vi "SubVI-AOMvolt-Power Calibration for 1064-PDver.vi"(3 "milliseconds to wait":u32=200, 4 "scan step #":dbl=25.0, 5 "Max voltage (V)":dbl=4.000000000000001, 6 "Min voltage (V)":dbl=0.5) -> (1 "Polynomial Coefficients":dbl[](array[numeric]) format="%0.2f", 2 "output cluster":T1)   [LabVIEW 2014]
uses:
  <vilib>/Analysis/baseanly.llb/Mean (DBL).vi
  <vilib>/Utility/file.llb/Write To Spreadsheet File (DBL).vi
  <vilib>/Analysis/NI_AALPro.lvlib
  <vilib>/Analysis/NI_AALBase.lvlib
panel:
  out "Cal-PD (mV)":dbl[](array[numeric])
  out "Cal-AOM (V)":dbl[](array[numeric])
  out "PD-AOM Graph":T2(graph)
  out "Voltage to AOM (V)":dbl
  out "Photodiode readout (mV)":dbl
  out "Scan size per step (V)":dbl=0.25
  in  "save cal curve?":bool
  # "**activate \ncontinuous power\ncontinuous AOM"
  # "continuous scaning power \nover AOM voltage range"
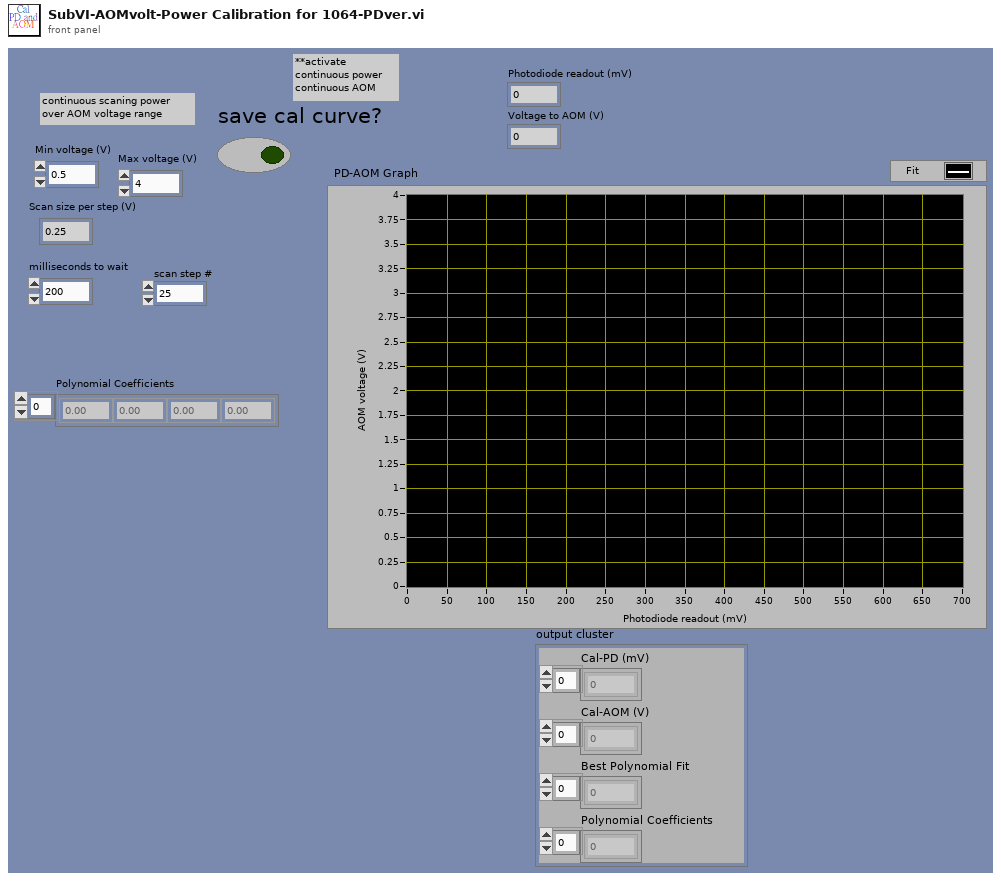
[diagram p1: front panel]
types:
  T1 = cluster{"Cal-PD (mV)":dbl[], "Cal-AOM (V)":dbl[], "Best Polynomial Fit":dbl[], "Polynomial Coefficients":dbl[]}
  T2 = cluster{"Cal-PD (mV)":dbl[], "Cal-AOM (V)":dbl[]}[]
  T3 = cluster{"Cal-PD (mV)":dbl[], "Best Polynomial Fit":dbl[]}
  T4 = cluster{"Cal-PD (mV)":dbl[], "Cal-AOM (V)":dbl[]}
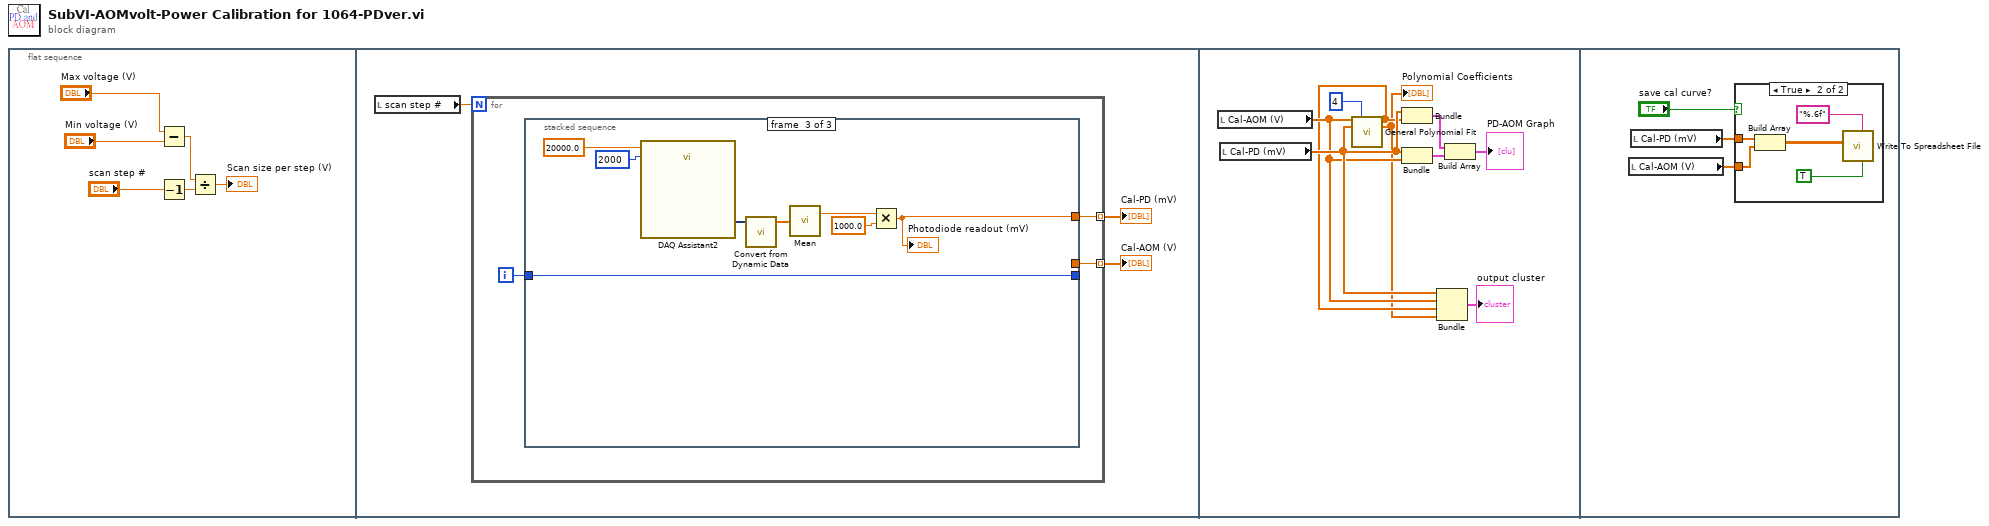
[diagram p0: block diagram]
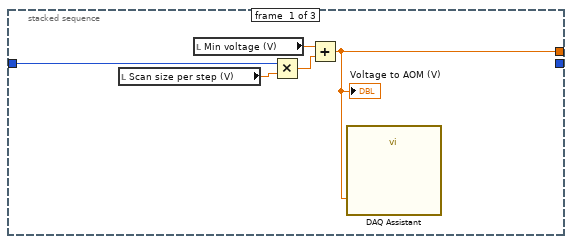
[diagram p2: hidden frame]
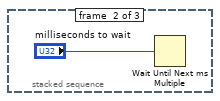
[diagram p3: hidden frame]
diagram:
  n1 = flat-sequence {
    frame #0 {
      n2 = Subtract(x="Max voltage (V)", y="Min voltage (V)") -> (x-y=w3:dbl)
      n3 = Decrement(x="scan step #") -> (x-1=w5:dbl)
      n4 = Divide(x=w3, y=w5) -> (x/y=→"Scan size per step (V)":dbl)
    }
    frame #1 {
      n5 = local read "scan step #"() -> (w9:dbl)
      n6 = for {
        N: w9 -> [_]
        tunnel: [w11] -> w7 mode=indexing
        tunnel: [w10] -> w8 mode=indexing
        i -> [w12]
        n7 = stacked-sequence {
          tunnel: w12 -> [w14 _ w26]
          tunnel: [_ _ w26] -> _
          tunnel: [_ _ w19] -> w11
          tunnel: [w17 _ _] -> w10
          frame #0 {
            n8 = local read "Scan size per step (V)"() -> (w15:dbl)
            n9 = local read "Min voltage (V)"() -> (w16:dbl)
            n10 = Multiply(x=w14, y=w15) -> (x*y=w13:dbl)
            n11 = Add(x=w16, y=w13) -> (x+y=w17:dbl)
            "Voltage to AOM (V)" <- w17
            n12 = call "DAQ Assistant"("data"=w17) -> ()  [unwired: 17 in, 2 out]
          }
          frame #1 {
            n13 = Wait Until Next ms Multiple(millisecond multiple="milliseconds to wait") -> ()  [unwired: 1 out]
          }
          frame #2 {
            n14 = call "DAQ Assistant2"("rate"=20000.0, "number of samples"=2000) -> ("data"=w24:dynamicdata)  [unwired: 15 in, 2 out]
            n15 = call "Convert from Dynamic Data"("Dynamic Data Type"=w24) -> ("Array"=w21:dbl[])  [unwired: 3 in]
            n16 = call-poly <vilib>:"Mean.vi"("X"=w21) -> ("mean"=w20:dbl)  [unwired: 1 out]
            n17 = Multiply(x=w20, y=1000.0) -> (x*y=w19:dbl)
            "Photodiode readout (mV)" <- w19
          }
        }
      }
      "Cal-AOM (V)" <- w8
      "Cal-PD (mV)" <- w7
    }
    frame #2 {
      n18 = local read "Cal-AOM (V)"() -> (w30:dbl[])
      n19 = local read "Cal-PD (mV)"() -> (w31:dbl[])
      n20 = call <vilib>:"General Polynomial Fit.vi"("Y"=w30, "polynomial order"=4, "X"=w31) -> ("Best Polynomial Fit"=w29:dbl[], "Polynomial Coefficients"=w28:dbl[])  [unwired: 9 in, 2 out]
      "Polynomial Coefficients" <- w28
      n21 = Bundle("Cal-PD (mV)"=w31, "Best Polynomial Fit"=w29) -> (w34:T3)  [unwired: 1 in]
      n22 = Bundle("Cal-PD (mV)"=w31, "Cal-AOM (V)"=w30) -> (w33:T4)  [unwired: 1 in]
      n23 = Bundle("Cal-PD (mV)"=w31, "Cal-AOM (V)"=w30, "Best Polynomial Fit"=w29, "Polynomial Coefficients"=w28) -> (→"output cluster":T1)  [unwired: 1 in]
      n24 = Build Array(w34, w33) -> (→"PD-AOM Graph":T2)
    }
    frame #3 {
      n25 = local read "Cal-AOM (V)"() -> (w36:dbl[])
      n26 = local read "Cal-PD (mV)"() -> (w37:dbl[])
      n27 = case shown="True" "save cal curve?" {
        tunnel: w37 -> [_ w42]
        tunnel: w36 -> [_ w41]
        frame False {
        }
        frame True {
          n28 = Build Array(w42, w41) -> (w40:dbl[][])
          n29 = call-poly <vilib>:"Write To Spreadsheet File.vi"("transpose? (no:F)"=TRUE, "format (%.3f)"="%.6f", "2D data"=w40) -> ()  [unwired: 3 in, 3 out]
        }
      }
    }
  }
